vi "Count Display Mode.vi"(7 "Read Value? (F)":bool, 8 "error in (no error)":errorcluster, 10 "Count Display Mode (Hold)":T1=enum."Hold", 11 "VISA resource name":refnum<visa-resource-name>) -> (0 "error out":errorcluster, 2 "Count Display Mode":T1=enum."Hold", 3 "VISA resource name out":refnum<visa-resource-name>)   [LabVIEW 2013, in "SRS SR400.lvlib"]
doc: "<B>SD { j }</B>\n\nIf j = 1, the SD command sets the count display mode to HOLD. If j = 0, the display mode will be CONTINUOUS. If j is absent, the display mode is returned."
uses:
  <instrlib>/SRS SR400/SRS SR400.lvlib
  <instrlib>/SRS SR400/Public/Typedefs/Count Display Mode.ctl
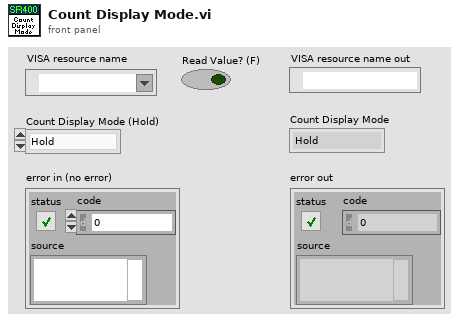
[diagram p1: front panel]
types:
  T1 = typedef "SRS SR400.lvlib/Count Display Mode.ctl" = enum16{"Continuous", "Hold"}
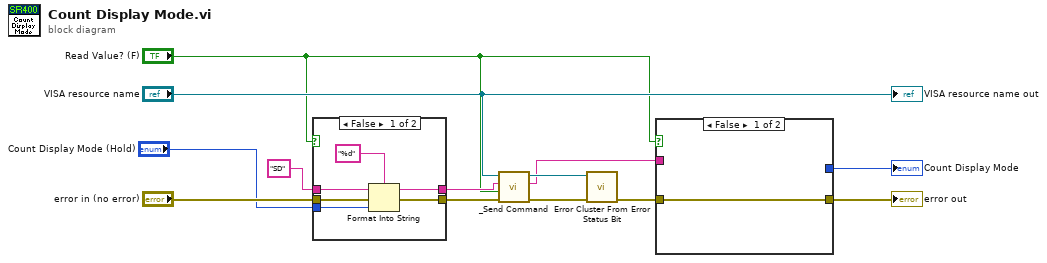
[diagram p0: block diagram]
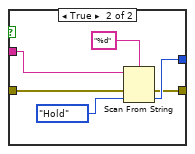
[diagram p2: hidden frame]
diagram:
  n1 = case shown="False" "Read Value? (F)" {
    tunnel: "error in (no error)" -> [w19 w20]
    tunnel: "SD" ("command") -> [w17 w21]
    tunnel: [w16 w21] -> w11
    tunnel: [w15 w20] -> w10
    tunnel: "Count Display Mode (Hold)" -> [w14 _]
    frame False {
      n2 = Format Into String(format string="%d", initial string=w17, error in=w19, w14) -> (resulting string=w16:string, error out=w15:errorcluster)
    }
    frame True {
    }
  }
  n3 = call <instrlib>:"_Send Command.vi"("error in (no error)"=w10, "Read Value? (F)"="Read Value? (F)", "Command"=w11, "VISA resource name"="VISA resource name") -> ("error out"=w6:errorcluster, "Response"=w3:string, "VISA resource name out"=w7:refnum<visa-resource-name>)  [unwired: 5 out]
  n4 = call <instrlib>:"Error Cluster From Error Status Bit.vi"("error in (no error)"=w6, "VISA resource name"=w7) -> ("error out"=w5:errorcluster)  [unwired: 8 in, 1 out]
  n5 = case shown="False" "Read Value? (F)" {
    tunnel: w5 -> [w22 w28]
    tunnel: w3 -> [_ w27]
    tunnel: [_ w25] -> w2
    tunnel: [w22 w23] -> w1
    frame False {
    }
    frame True {
      n6 = Scan From String(format string="%d", input string=w27, error in=w28, default 1=Count_Display_Mode."Hold" ("Count Display Mode (Hold)")) -> (error out=w23:errorcluster, output 1=w25:T1)  [unwired: 1 in, 2 out]
    }
  }
  "error out" <- w1
  "Count Display Mode" <- w2
  "VISA resource name out" <- "VISA resource name"
